vi "Blink when valuechange subvi.vi"(9 "Indicator or ctrl to look up value change":refnum<vi>) -> (2 "Elapsed Time (s)":dbl caption="Verstrichene Zeit (s)", 3 "Blinkend":bool)   [LabVIEW 2016]
uses:
  <userlib>/_OpenG.lib/comparison/comparison.llb/Variant Changed__ogtk.vi
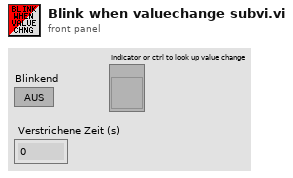
[diagram p1: front panel]
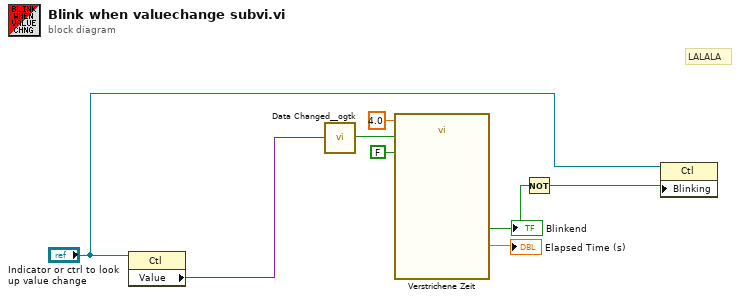
[diagram p0: block diagram]
diagram:
  # "LALALA"
  n1 = property class="Ctl"(reference="Indicator or ctrl to look up value change") -> ("Value"=w2:variant)  [unwired: 1 in, 2 out]
  n2 = call-poly <userlib>:"Data Changed__ogtk.vi"("Variant"=w2) -> ("Changed"=w3:bool)
  n3 = call "Verstrichene Zeit"("Time Target (s)"=4.0, "Reset"=w3, "Auto Reset"=FALSE) -> ("Elapsed Time (s)"=→"Elapsed Time (s)":dbl, "Time has Elapsed"=w8:bool)  [unwired: 9 in, 6 out]
  "Blinkend" <- w8
  n4 = Not(x=w8) -> (.not. x?=w7:bool)
  n5 = property class="Ctl"(reference="Indicator or ctrl to look up value change", "Blinking"=w7) -> ()  [unwired: 1 in, 2 out]
